vi "CIMAQ_Skeleton_Endpoints.vi"(10 "Endpoints dst":T1, 11 "Skeleton in":T1) -> (3 "Endpoints":T1)   [LabVIEW 2017]
uses:
  <vilib>/vision/Image Controls.llb/IMAQ Image.ctl
  <vilib>/vision/NI_Vision_Development_Module.lvlib
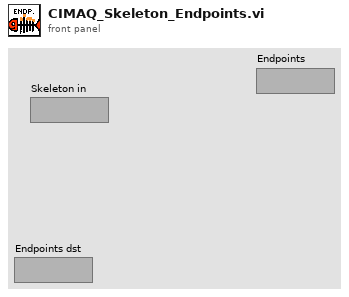
[diagram p1: front panel]
types:
  T1 = typedef "IMAQ Image.ctl" = refnum<image>
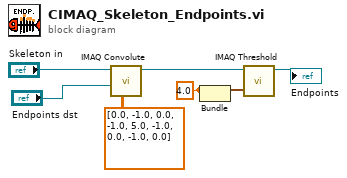
[diagram p0: block diagram]
diagram:
  w5 = sgl 4.0 ("Constant")
  n1 = call "IMAQ Convolute"("Kernel"=sgl[][] [[0.0, -1.0, 0.0], [-1.0, 5.0, -1.0], [0.0, -1.0, 0.0]], "Image Dst"="Endpoints dst", "Image Src"="Skeleton in") -> ("Image Dst Out"=w1:T1)  [unwired: 4 in, 4 out]
  n2 = Bundle("Constant"=w5, "Constant"=w5) -> (w4:cluster{"Constant":sgl, "Constant":sgl})  [unwired: 1 in]
  n3 = call "IMAQ Threshold"("Range"=w4, "Image Src"=w1) -> ("Image Dst Out"=→"Endpoints":T1)  [unwired: 8 in, 1 out]
